vi "Iteration Counter.vi"() -> ()   [LabVIEW 2019]
panel:
  in  "Counter":dbl
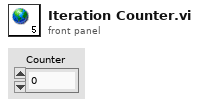
[diagram p1: front panel]
diagram:
